vi "6. CoersionDot.vi"() -> ()   [LabVIEW 2019]
panel:
  out "u8 Ind 2":u8
  out "u16 Ind":u16
  out "u8 Ind":u8
  in  "u16Ctl":u16
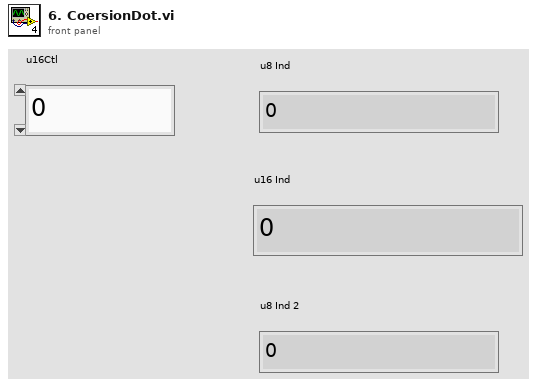
[diagram p1: front panel]
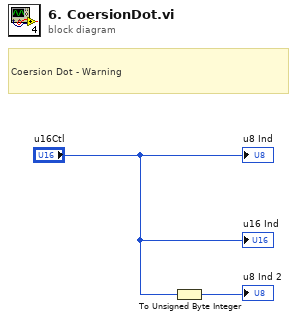
[diagram p0: block diagram]
diagram:
  # "Coersion Dot - Warning"
  n1 = To Unsigned Byte Integer(number="u16Ctl") -> (unsigned 8bit integer=→"u8 Ind 2":u8)
  "u8 Ind" <- "u16Ctl"
  "u16 Ind" <- "u16Ctl"
